vi "X-Axis into Resolution.vi"(0 "X-axis (nm)":dbl[](array[numeric])=[571.2504622529284, 585.6489231225254, 600.0000000000001, 614.300024178551, 628.5453659653462] format="%.4f") -> (1 "Res/nm/20µ":dbl=25.810711007261716 format="%.4f", 2 "Res/nm/100µ":dbl=25.810711007261716 format="%.4f", 3 "Res/nm/500µ":dbl=25.810711007261716 format="%.4f", 4 "Res/meV/20µ":dbl=25.810711007261716 format="%.4f", 8 "Res/meV/100µ":dbl=25.810711007261716 format="%.4f", 12 "Res/cm-1/20µ":dbl=25.810711007261716 format="%.4f", 13 "Res/cm-1/100µ":dbl=25.810711007261716 format="%.4f", 14 "Res/cm-1/500µ":dbl=25.810711007261716 format="%.4f", 15 "Res/meV/500":dbl=25.810711007261716 format="%.4f")   [LabVIEW 2025]
doc: "Author: Scott Hannahs <sth@magnet.fsu.edu>\n\nThis software is licensed for use under the “MIT License\"\nCopyright (c) 2025 Scott Hannahs, sth@sth@magnet.sthnet.net\n\nPermission is hereby granted, free of charge, to any person obtaining a copy of this software and associated documentation files (the \"Software\"), to deal in the Software without restriction, including without limitation the rights to use, copy, modify, merge, publish, distribute, sublicense, and/or sell copies of the Software, and to permit persons to whom the Software is furnished to do so, subject to the following conditions: The above copyright notice and this permission notice shall be included in all copies or substantial portions of the Software.\n\nTHE SOFTWARE IS PROVIDED \"AS IS\", WITHOUT WARRANTY OF ANY KIND, EXPRESS OR IMPLIED, INCLUDING BUT NOT LIMITED TO THE WARRANTIES OF MERCHANTABILITY, FITNESS FOR A PARTICULAR PURPOSE AND NONINFRINGEMENT. IN NO EVENT SHALL THE AUTHORS OR COPYRIGHT HOLDERS BE LIABLE FOR ANY CLAIM, DAMAGES OR OTHER LIABILITY, WHETHER IN AN ACTION OF CONTRACT, TORT OR OTHERWISE, ARISING FROM, OUT OF OR IN CONNECTION WITH THE SOFTWARE OR THE USE OR OTHER DEALINGS IN THE SOFTWARE."
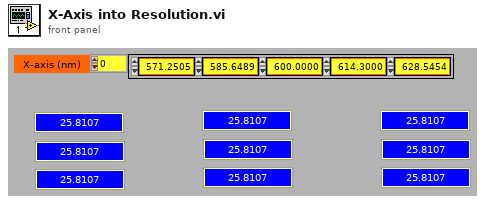
[diagram p1: front panel]
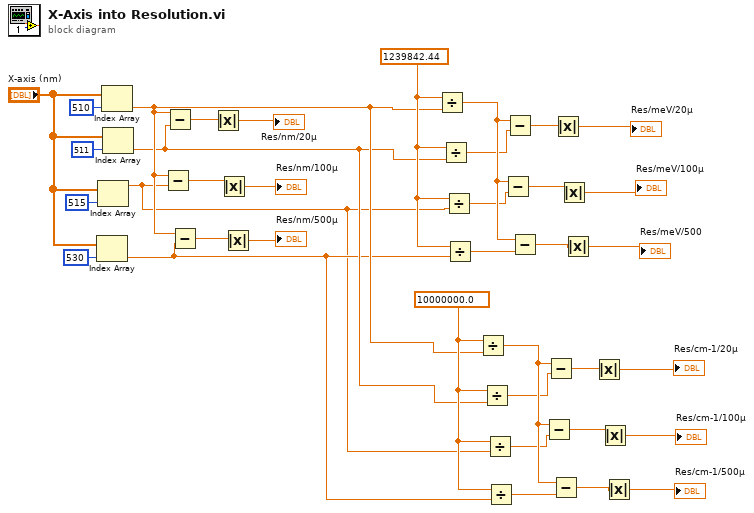
[diagram p0: block diagram]
diagram:
  w12 = 10000000.0 ("Index")
  w23 = 1239842.44 ("Index")
  n1 = Index Array(array="X-axis (nm)", index=530 ("Index")) -> (element=w5:dbl)
  n2 = Index Array(array="X-axis (nm)", index=515 ("Index")) -> (element=w1:dbl)
  n3 = Index Array(array="X-axis (nm)", index=510 ("Index")) -> (element=w7:dbl)
  n4 = Index Array(array="X-axis (nm)", index=511 ("Index")) -> (element=w6:dbl)
  n5 = Subtract(x=w7, y=w1) -> (x-y=w31:dbl)
  n6 = Subtract(x=w7, y=w6) -> (x-y=w32:dbl)
  n7 = Subtract(x=w7, y=w5) -> (x-y=w30:dbl)
  n8 = Absolute Value(x=w32) -> (abs(x)=→"Res/nm/20µ":dbl)
  n9 = Absolute Value(x=w31) -> (abs(x)=→"Res/nm/100µ":dbl)
  n10 = Absolute Value(x=w30) -> (abs(x)=→"Res/nm/500µ":dbl)
  n11 = Divide(x=w23, y=w7) -> (x/y=w22:dbl)
  n12 = Divide(x=w23, y=w6) -> (x/y=w21:dbl)
  n13 = Divide(x=w23, y=w1) -> (x/y=w20:dbl)
  n14 = Divide(x=w23, y=w5) -> (x/y=w19:dbl)
  n15 = Divide(x=w12, y=w7) -> (x/y=w11:dbl)
  n16 = Divide(x=w12, y=w6) -> (x/y=w10:dbl)
  n17 = Divide(x=w12, y=w1) -> (x/y=w9:dbl)
  n18 = Divide(x=w12, y=w5) -> (x/y=w8:dbl)
  n19 = Subtract(x=w22, y=w20) -> (x-y=w25:dbl)
  n20 = Subtract(x=w22, y=w21) -> (x-y=w26:dbl)
  n21 = Subtract(x=w22, y=w19) -> (x-y=w24:dbl)
  n22 = Subtract(x=w11, y=w9) -> (x-y=w14:dbl)
  n23 = Subtract(x=w11, y=w10) -> (x-y=w15:dbl)
  n24 = Subtract(x=w11, y=w8) -> (x-y=w13:dbl)
  n25 = Absolute Value(x=w26) -> (abs(x)=→"Res/meV/20µ":dbl)
  n26 = Absolute Value(x=w25) -> (abs(x)=→"Res/meV/100µ":dbl)
  n27 = Absolute Value(x=w24) -> (abs(x)=→"Res/meV/500":dbl)
  n28 = Absolute Value(x=w15) -> (abs(x)=→"Res/cm-1/20µ":dbl)
  n29 = Absolute Value(x=w14) -> (abs(x)=→"Res/cm-1/100µ":dbl)
  n30 = Absolute Value(x=w13) -> (abs(x)=→"Res/cm-1/500µ":dbl)
